vi "selection sorting.vi"(2 "values between 1~10000":dbl[](array[numeric]), 4 "N numbers":i32) -> ()   [LabVIEW 2014]
panel:
  out "Waveform Graph":dbl[](graph)
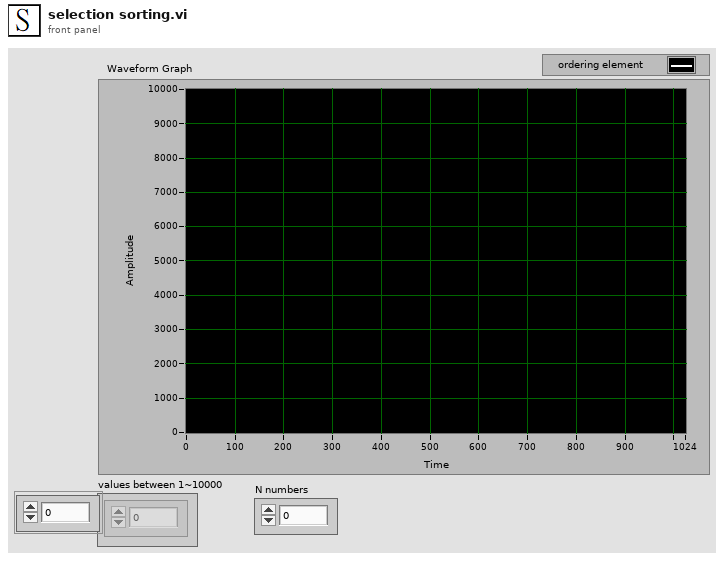
[diagram p1: front panel]
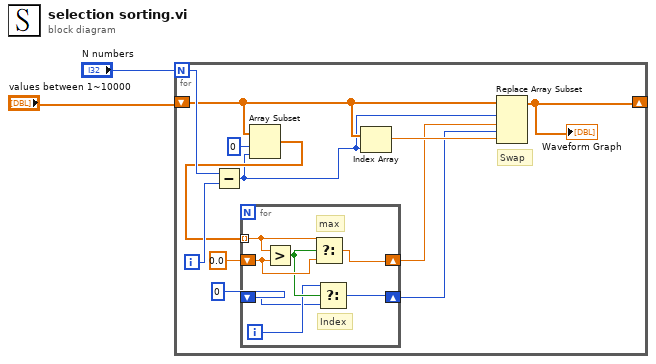
[diagram p0: block diagram]
diagram:
  n1 = for {
    N: "N numbers" -> [w13]
    shift-right: [w3] -> _
    shift-left: "values between 1~10000" -> [w11]
    i -> [w12]
    # "Swap"
    n2 = Subtract(x=w13, y=w12) -> (x-y=w4:i32)
    n3 = Array Subset(array=w11, index=0, length=w4) -> (w9:dbl[])
    n4 = for {
      tunnel: w9 -> [w21] mode=indexing
      shift-right: [w19] -> w6
      shift-left: 0.0 -> [w20]
      shift-right: [w18] -> w5
      shift-left: 0 -> [w15]
      i -> [w16]
      # "Index"
      # "max"
      n5 = Greater?(x=w21, y=w20) -> (0:w17:bool)
      n6 = Select(t=w21, s=w17, f=w20) -> (s? t:f=w19:dbl)
      n7 = Select(t=w16, s=w17, f=w15) -> (s? t:f=w18:i32)
    }
    n8 = Index Array(array=w11, index=w4) -> (element=w10:dbl)
    n9 = Replace Array Subset(array=w11, new element #1=w6, index #1=w4, new element #2=w10, index #2=w5) -> (w3:dbl[])
    "Waveform Graph" <- w3
  }
